vi "Store_Missed_Events.vi"(0 "LabVIEW Web Service Request":refnum<class "Web Request.lvclass">, 1 "deltaArray":dbl[][](array[numeric]), 2 "variablePath":string[][](array[string]), 3 "variableArray":string[][](array[string]), 5 "expId":string, 7 "initTime":u32, 9 "variables":string, 11 "arraylength":i32, 12 "expIndex":i32, 13 "inputArray":dbl[](array[numeric]), 15 "userIndex":i32) -> (4 "LabVIEW Web Service Request out":refnum<class "Web Request.lvclass">, 6 "path":path)   [LabVIEW 2020]
doc: "Waits for the client to reconnect and stores all missed events"
uses:
  <vilib>/wsapi/Web Request.lvclass
  Configuration/Global_Configurations.vi
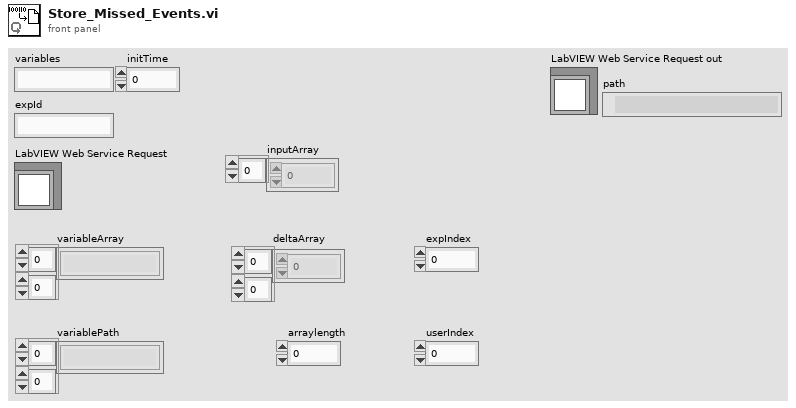
[diagram p1: front panel]
types:
  T1 = cluster{"Path":path, "Name":string, "Authors":string, "Keywords":string, "Description":string, "Cameras":cluster{"Base URL":string, "Path":string, "Name":string}[], "Sampling":cluster{"Sampled Variable":string, "Delta":dbl}[], "Sampling Freq":u32}[]
  T2 = cluster{"Path":path, "Name":string, "Authors":string, "Keywords":string, "Description":string, "Cameras":cluster{"Base URL":string, "Path":string, "Name":string}[], "Sampling":cluster{"Sampled Variable":string, "Delta":dbl}[], "Sampling Freq":u32}
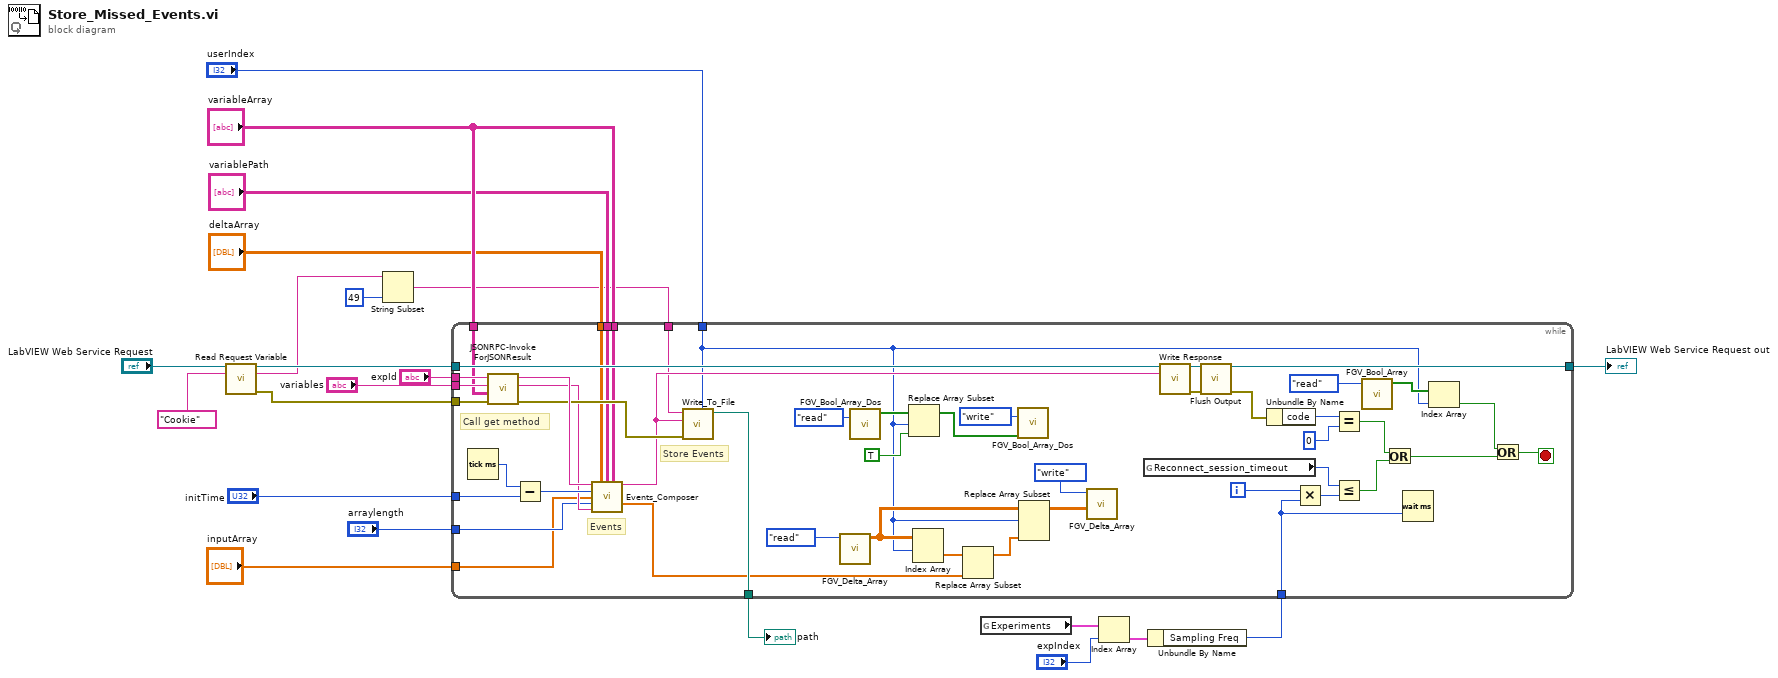
[diagram p0: block diagram]
diagram:
  n1 = call <vilib>:"Read Request Variable.vi"("LabVIEW Web Service Request"="LabVIEW Web Service Request", "variable name"="Cookie") -> ("LabVIEW Web Service Request out"=w17:refnum<class "Web Request.lvclass">, "value"=w4:string, "error out"=w16:errorcluster)  [unwired: 11 in]
  n2 = String Subset(string=w4, length (rest)=49) -> (substring=w3:string)  [unwired: 1 in]
  n3 = global read "Global_Configurations.vi" "Experiments"() -> (w10:T1)
  n4 = Index Array(array=w10, index="expIndex") -> (element=w9:T2)
  n5 = Unbundle By Name(w9) -> ("Sampling Freq"=w7:u32)
  n6 = while {
    tunnel: w17 -> [w53]
    tunnel: "expId" -> [w67]
    tunnel: "initTime" -> [w64]
    tunnel: [w63] -> w19
    tunnel: "variables" -> [w61]
    tunnel: w16 -> [w55]
    tunnel: [w54] -> w15
    tunnel: "arraylength" -> [w48]
    tunnel: "variableArray" -> [w47]
    tunnel: "variableArray" -> [w46]
    tunnel: "deltaArray" -> [w45]
    tunnel: "variablePath" -> [w44]
    tunnel: w7 -> [w40]
    tunnel: w3 -> [w39]
    tunnel: "userIndex" -> [w23]
    tunnel: "inputArray" -> [w36]
    i -> [w58]
    stop <- w41 stop-if-true
    # "Store Events"
    # "Events"
    # "Call get method"
    n7 = Tick Count (ms)() -> (millisecond timer value=w65:u32)
    n8 = call "JSONRPC-InvokeForJSONResult.vi"("error in"=w55, "variableArray"=w47, "variables"=w61, "expid"=w67) -> ("error out"=w52:errorcluster, "responseper"=w49:string, "response"=w66:string)  [unwired: 5 in]
    n9 = Subtract(x=w65, y=w64) -> (x-y=w60:u32)
    n10 = call "Events_Composer.vi"("responsein"=w66, "deltaArray"=w45, "path"=w44, "variableArray"=w46, "time"=w60, "inputArray"=w36, "arraylength"=w48, "responseper"=w49) -> ("responseout"=w51:string, "outputArray"=w29:dbl[])  [unwired: 6 in]
    n11 = call "Write_To_File.vi"("userIndex"=w23, "error in"=w52, "data"=w51, "cookie"=w39) -> ("path"=w54:path)  [unwired: 6 in, 1 out]
    n12 = call "FGV_Delta_Array.vi"("Enum"=enum16{"read", "write"}."read" ("operation (0:open)")) -> ("array out"=w33:dbl[][])  [unwired: 10 in]
    n13 = call "FGV_Bool_Array_Dos.vi"("Enum"=enum16{"read", "write"}."read" ("operation (0:open)")) -> ("Array Out"=w27:bool[])  [unwired: 10 in]
    n14 = Replace Array Subset(array=w27, new element=TRUE, index=w23) -> (w28:bool[])
    n15 = Index Array(array=w33, index (row)=w23) -> (element=w35:dbl[])  [unwired: 1 in]
    n16 = Replace Array Subset(array=w35, new element=w29) -> (w34:dbl[])  [unwired: 1 in]
    n17 = call "FGV_Bool_Array_Dos.vi"("Array In"=w28, "Enum"=enum16{"read", "write"}."write" ("operation (0:open)")) -> ()  [unwired: 9 in, 1 out]
    n18 = Replace Array Subset(array=w33, new element=w34, index (row)=w23) -> (w32:dbl[][])  [unwired: 1 in]
    n19 = call "FGV_Delta_Array.vi"("array in"=w32, "Enum"=enum16{"read", "write"}."write" ("operation (0:open)")) -> ()  [unwired: 9 in, 1 out]
    n20 = global read "Global_Configurations.vi" "Reconnect_session_timeout"() -> (w57:u32)
    n21 = call <vilib>:"Write Response.vi"("LabVIEW Web Service Request"=w53, "response string"=w51) -> ("LabVIEW Web Service Request out"=w70:refnum<class "Web Request.lvclass">, "error out"=w71:errorcluster)  [unwired: 12 in]
    n22 = call <vilib>:"Flush Output.vi"("LabVIEW Web Service Request"=w70, "error in (no error)"=w71) -> ("LabVIEW Web Service Request out"=w63:refnum<class "Web Request.lvclass">, "error out"=w62:errorcluster)  [unwired: 12 in]
    n23 = Unbundle By Name(w62) -> ("code"=w69:i32)
    n24 = Multiply(x=w58, y=w40) -> (x*y=w59:u32)
    n25 = Equal?(x=w69, y=0) -> (x = y?=w50:bool)
    n26 = Less Or Equal?(x=w57, y=w59) -> (x <= y?=w56:bool)
    n27 = call "FGV_Bool_Array.vi"("Enum"=enum16{"read", "write"}."read" ("operation (0:open)")) -> ("Array Out"=w38:bool[])  [unwired: 10 in]
    n28 = Or(x=w50, y=w56) -> (x .or. y?=w42:bool)
    n29 = Wait (ms)(milliseconds to wait=w40) -> ()  [unwired: 1 out]
    n30 = Index Array(array=w38, index=w23) -> (element=w37:bool)
    n31 = Or(x=w37, y=w42) -> (x .or. y?=w41:bool)
  }
  "LabVIEW Web Service Request out" <- w19
  "path" <- w15
